vi "Open_eID_Image.vi"(11 "eID":T2) -> (3 "image data":T1)   [LabVIEW 2020]
uses:
  Controls/User_DB.ctl
  <vilib>/picture/picture.llb/imagedata.ctl
panel:
  out "Array":string[](array[string])
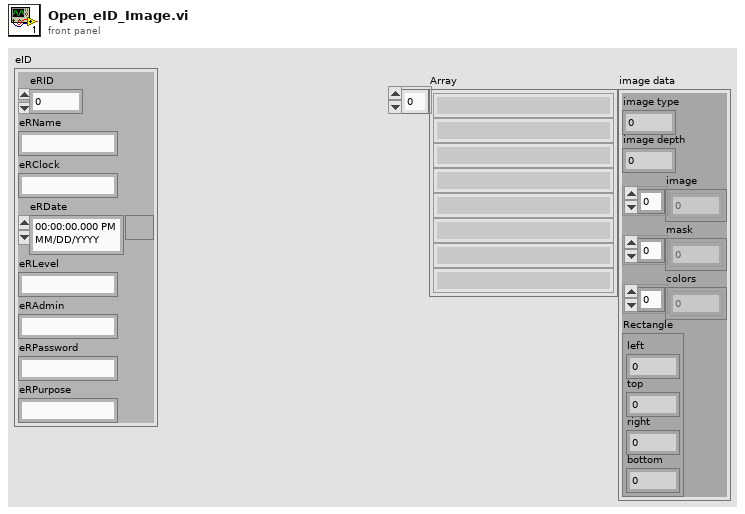
[diagram p1: front panel]
types:
  T1 = typedef "imagedata.ctl" = cluster{"image type":i32, "image depth":i32, "image":u8[], "mask":u8[], "colors":u32[], "Rectangle":cluster{"left":i16, "top":i16, "right":i16, "bottom":i16}}
  T2 = typedef "User_DB.ctl" = cluster{"eRID":u16, "eRName":string, "eRClock":string, "eRDate":timestamp, "eRLevel":string, "eRAdmin":string, "eRPassword":string, "eRPurpose":string}
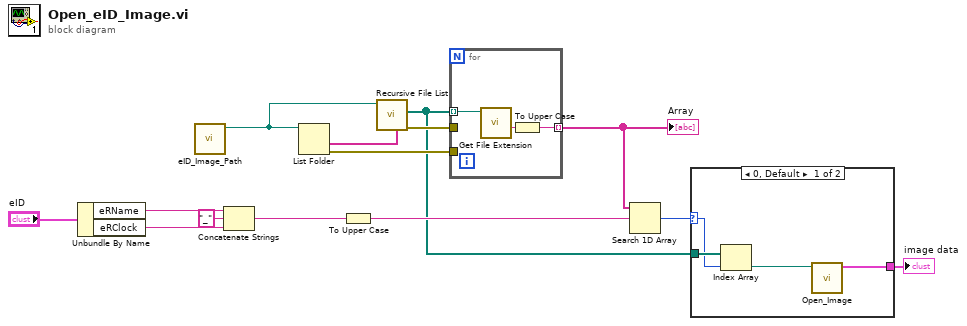
[diagram p0: block diagram]
diagram:
  n1 = Unbundle By Name("eID") -> ("eRName"=w14:string, "eRClock"=w13:string)
  n2 = call "eID_Image_Path.vi"() -> ("Path out"=w10:path)  [unwired: 11 in]
  n3 = Concatenate Strings(w14, "_" ("string"), w13) -> (w6:string)
  n4 = List Folder(path=w10) -> (folder names=w9:string[], error out=w8:errorcluster)  [unwired: 3 in, 2 out]
  n5 = To Upper Case(1:w6) -> (0:w4:string)
  n6 = call <vilib>:"Recursive File List.vi"("Folders to Exclude"=w9, "Folder Path"=w10) -> ("error out"=w7:errorcluster, "All Files in Dir"=w2:path[])  [unwired: 5 in, 3 out]
  n7 = for {
    tunnel: w8 -> [_]
    tunnel: w7 -> [_]
    tunnel: w2 -> [w17] mode=indexing
    tunnel: [w15] -> w5 mode=indexing
    n8 = call <vilib>:"Get File Extension.vi"("file"=w17) -> ("filename without extension"=w16:string)  [unwired: 6 in, 4 out]
    n9 = To Upper Case(1:w16) -> (0:w15:string)
  }
  "Array" <- w5
  n10 = Search 1D Array(1D array=w5, element=w4) -> (index of element=w3:i32)  [unwired: 1 in]
  n11 = case shown="0, Default" w3 {
    selector: w3 -> [w20 _]
    tunnel: w2 -> [w21 _]
    tunnel: [w18 _] -> w1
    frame 0, Default {
      n12 = Index Array(array=w21, index=w20) -> (element=w19:path)
      n13 = call "Open_Image.vi"("NewVal"=w19) -> ("image data"=w18:T1)  [unwired: 10 in]
    }
    frame -1 {
    }
  }
  "image data" <- w1
